vi "OPC UA Writer.vi"(8 "Temperature":dbl, 10 "Node ID C":string="ns=2;s=Temperature", 11 "Server Endpoint URL":string="opc.tcp://LAPTOP-UEHKTQQC:49580") -> ()   [LabVIEW 2019]
uses:
  <vilib>/OPCUA/controls/NodeId.ctl
  <vilib>/OPCUA/controls/Write Status.ctl
  <vilib>/OPCUA/client/Multiple Write Double.vi
  <vilib>/OPCUA/NI OPC UA Client.lvlib
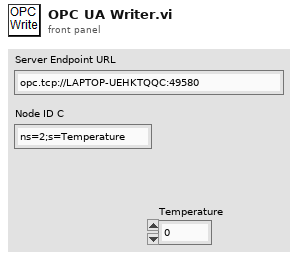
[diagram p1: front panel]
types:
  T1 = cluster{"message mode":enum16{"None", "Sign", "Sign and Encrypt"}, "security":enum16{"Basic256", "Basic128Rsa15"}}
  T2 = typedef "NodeId.ctl" = string
  T3 = typedef "Write Status.ctl" = u32
  T4 = cluster{"node ID":T2, "value":dbl, "timestamp (current time)":timestamp, "node status":T3}
  T5 = typedef "OPC UA Client Refnum.ctl" = refnum<k21>
  T6 = cluster{"node ID":T2, "value":dbl, "timestamp (current time)":timestamp, "node status":T3}[]
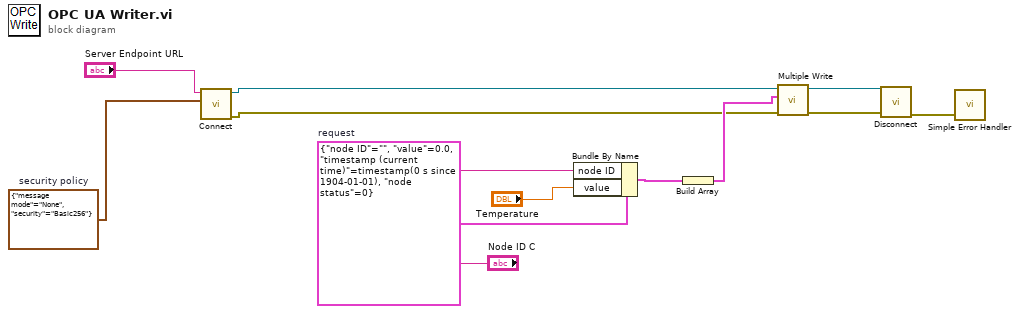
[diagram p0: block diagram]
diagram:
  w4 = T1 {"message mode"=enum."None", "security"=enum."Basic256"}  # security policy
  w9 = T4 {"node ID"="", "value"=0.0, "timestamp (current time)"=timestamp(0 s since 1904-01-01), "node status"=0}  # request
  n1 = call <vilib>:"Connect.vi"("security policy"=w4, "server endpoint URL"="Server Endpoint URL") -> ("error out"=w5:errorcluster, "OPC UA client refnum out"=w6:T5)  [unwired: 7 in, 1 out]
  n2 = Bundle By Name "Bundle By Name"(cluster=w9, "node ID"="Node ID C", "value"="Temperature") -> (w8:T4)
  n3 = Build Array "Build Array"(w8) -> (w7:T6)
  n4 = call-poly <vilib>:"Multiple Write.vi"("error in (no error)"=w5, "requests"=w7, "OPC UA client refnum in"=w6) -> ("error out"=w2:errorcluster, "OPC UA client refnum out"=w3:T5)  [unwired: 5 in, 2 out]
  n5 = call <vilib>:"Disconnect.vi"("error in (no error)"=w2, "OPC UA client refnum in"=w3) -> ("error out"=w11:errorcluster)  [unwired: 9 in]
  n6 = call <vilib>:"Simple Error Handler.vi"("error in (no error)"=w11) -> ()  [unwired: 4 in, 5 out]
